vi "pulse_distribute_tester.vi"() -> ()   [LabVIEW 2021]
uses:
  <instrlib>/_niInstr/Basic Elements/v1/FPGA/niInstr Basic Elements v1 FPGA.lvlib
  <instrlib>/_niInstr/Basic Elements/v1/FPGA/Private/Count Up U64.vi
  CTL/mode_type.ctl
  pdw.ctl
  <instrlib>/_niInstr/DSP/v1/Shared/Public/IQ Data.ctl
  <instrlib>/_niInstr/DSP/v1/Shared/niInstr DSP v1 Shared.lvlib
panel:
  in  "bigger then":i32
  in  "num of loops":i32
  out "Waveform Graph":i16[][](graph)
  out "pulses read":u64=36
  in  "stop":bool
  out "output cluster":T1 {"I" format="%#_6f"}
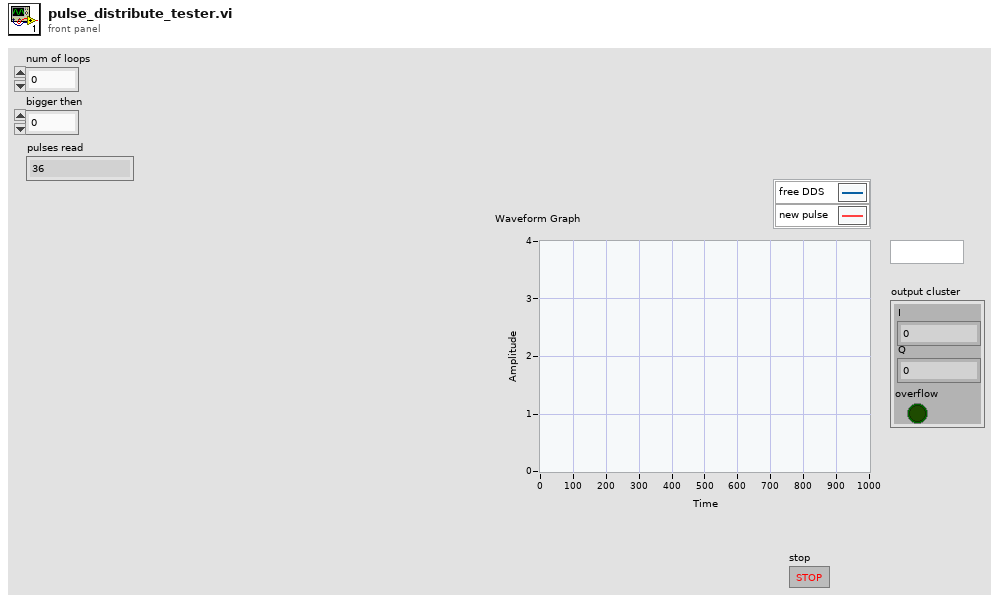
[diagram p1: front panel]
types:
  T1 = typedef "niInstr DSP v1 Shared.lvlib/IQ Data.ctl" = cluster{"I":fxp<+/-,18,1>, "Q":fxp<+/-,18,1>, "overflow":bool}
  T2 = typedef "pdw.ctl" = cluster{"PW":u32, "frequency shift":fxp<+/-,48,0>, "amp":fxp<+/-,18,1>, "mode type":T3, "mode depth":u32, "mode filter":u8, "phase shift":fxp<+/-,16,1>, "pulse shape filter":u8}
  T3 = typedef "mode_type.ctl" = enum8{"CW", "NC - CW", "NC - cw", "LFM", "BPSK", "QPSK"}
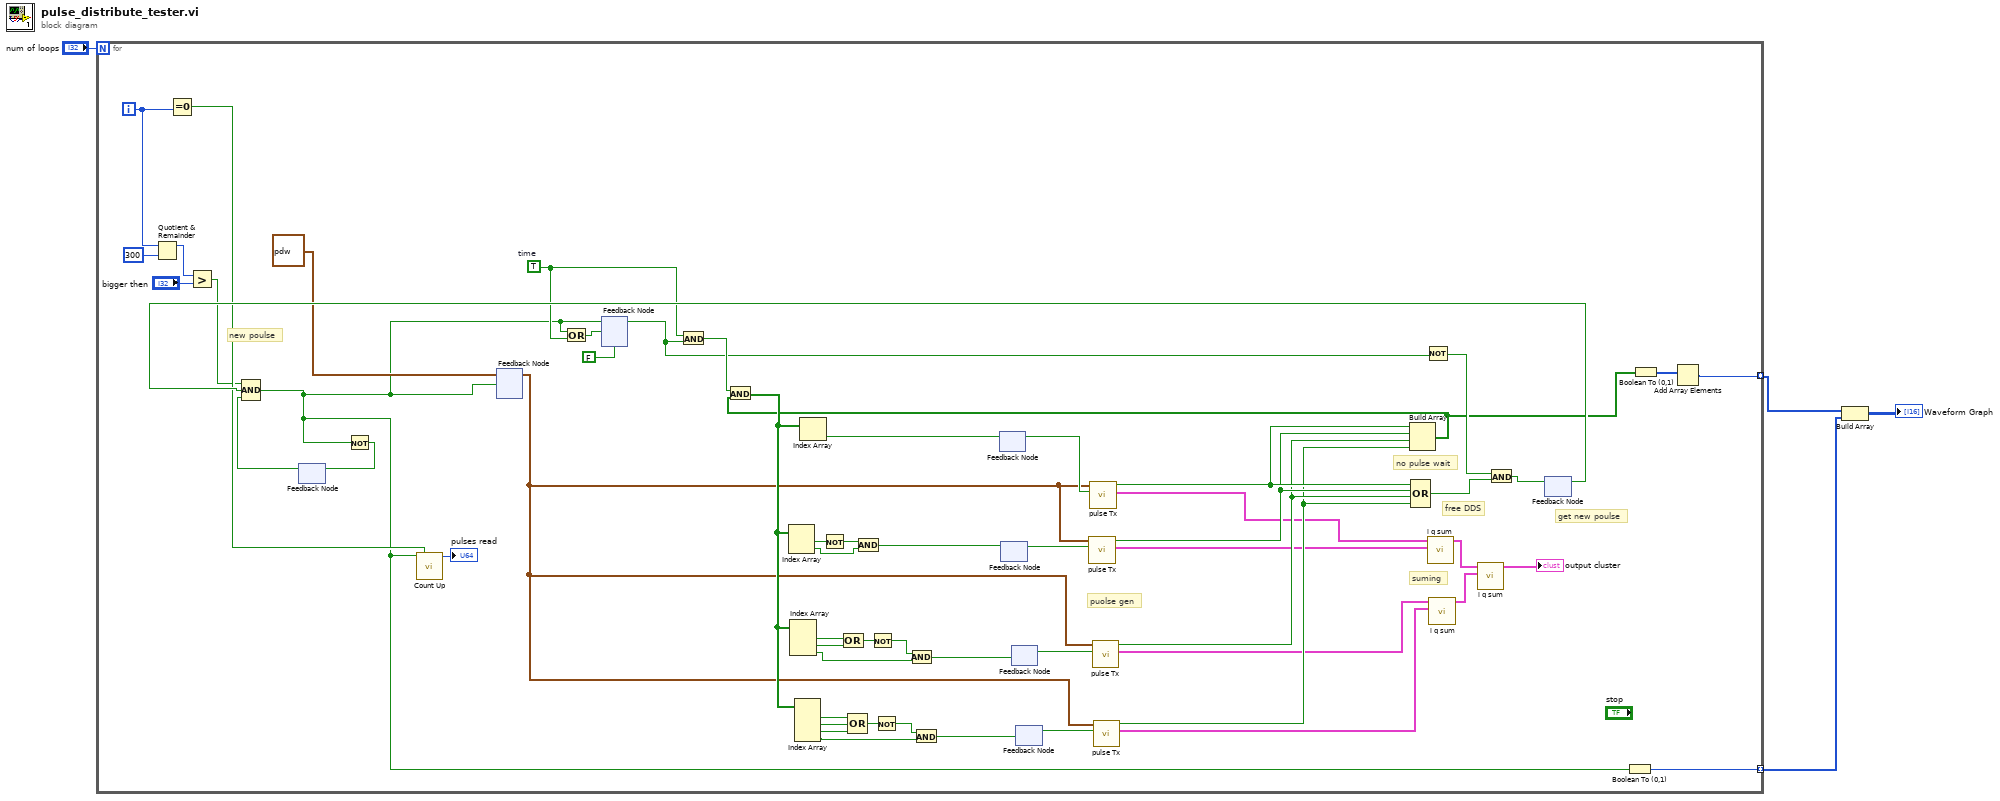
[diagram p0: block diagram]
diagram:
  n1 = for {
    N: "num of loops" -> [_]
    tunnel: [w13] -> w3 mode=indexing
    tunnel: [w10] -> w4 mode=indexing
    i -> [w9]
    w18 = TRUE  # time
    # "new poulse"
    # "suming"
    # "puolse gen"
    # "get new poulse"
    # "no pulse wait"
    # "free DDS"
    n2 = Quotient & Remainder(x=w9, y=300) -> (x-y*floor(x/y)=w7:i32)  [unwired: 1 out]
    n3 = Equal To 0?(x=w9) -> (x = 0?=w21:bool)
    n4 = Greater?(x=w7, y="bigger then") -> (0:w5:bool)
    n5 = feedback #1() -> (w23:bool)  [unwired: 1 in]
    n6 = feedback #2() -> (w15:T2)  [unwired: 1 in]
    n7 = feedback #3(FALSE ("Output Valid")) -> (w17:bool)
    n8 = And(x=w18, y=w17) -> (x .and. y?=w42:bool)
    n9 = feedback #4() -> (w31:bool)  [unwired: 1 in]
    n10 = feedback #5() -> (w53:bool)  [unwired: 1 in]
    n11 = feedback #6() -> (w52:bool)  [unwired: 1 in]
    n12 = feedback #7() -> (w50:bool)  [unwired: 1 in]
    n13 = call "pulse Tx.vi"("take it!"=w53, "Cluster"=w15) -> ("data out"=w37:T1, "free dds"=w62:bool)  [unwired: 5 in, 3 out]
    n14 = call "pulse Tx.vi"("take it!"=w31, "Cluster"=w15) -> ("data out"=w38:T1, "free dds"=w63:bool)  [unwired: 5 in, 3 out]
    n15 = call "pulse Tx.vi"("take it!"=w52, "Cluster"=w15) -> ("data out"=w36:T1, "free dds"=w51:bool)  [unwired: 5 in, 3 out]
    n16 = call "pulse Tx.vi"("take it!"=w50, "Cluster"=w15) -> ("data out"=w35:T1, "free dds"=w43:bool)  [unwired: 5 in, 3 out]
    n17 = Build Array(w63, w62, w51, w43) -> (w12:bool[])
    n18 = And(x=w42, y=w12) -> (x .and. y?=w41:bool[])
    n19 = Index Array(array=w41) -> (element #1=w61:bool, element #2=w59:bool)  [unwired: 2 in]
    n20 = Index Array(array=w41) -> (element #1=w55:bool, element #2=w56:bool, element #3=w57:bool)  [unwired: 3 in]
    n21 = Index Array(array=w41) -> (element #1=w48:bool, element #2=w47:bool, element #3=w44:bool, element #4=w45:bool)  [unwired: 4 in]
    n22 = Index Array(array=w41) -> (element=w29:bool)  [unwired: 1 in]
    n23 = Not(x=w61) -> (.not. x?=w60:bool)
    n24 = Compound Arithmetic op=OR(w55, w56) -> (w54:bool)
    n25 = Compound Arithmetic op=OR(w48, w47, w44) -> (w49:bool)
    n26 = And(x=w60, y=w59) -> (x .and. y?=w28:bool)
    n27 = Not(x=w54) -> (.not. x?=w58:bool)
    n28 = Not(x=w49) -> (.not. x?=w46:bool)
    n29 = And(x=w58, y=w57) -> (x .and. y?=w27:bool)
    n30 = And(x=w46, y=w45) -> (x .and. y?=w26:bool)
    n31 = feedback-in #4(w29) -> ()
    n32 = feedback-in #5(w28) -> ()
    n33 = feedback-in #6(w27) -> ()
    n34 = feedback-in #7(w26) -> ()
    n35 = Compound Arithmetic op=OR(w63, w62, w51, w43) -> (w39:bool)
    n36 = Not(x=w17) -> (.not. x?=w40:bool)
    n37 = call "i q sum.vi"(10:"data in"=w37, 11:"data in"=w38) -> ("output cluster"=w34:T1)  [unwired: 8 in, 1 out]
    n38 = call "i q sum.vi"(10:"data in"=w35, 11:"data in"=w36) -> ("output cluster"=w33:T1)  [unwired: 8 in, 1 out]
    n39 = call "i q sum.vi"(10:"data in"=w33, 11:"data in"=w34) -> ("output cluster"=→"output cluster":T1)  [unwired: 8 in, 1 out]
    n40 = And(x=w40, y=w39) -> (x .and. y?=w30:bool)
    n41 = feedback-in #8(w30) -> ()
    n42 = feedback #8() -> (w24:bool)  [unwired: 1 in]
    n43 = Compound Arithmetic op=AND(w5, w24, w23) -> (w14:bool)
    n44 = Not(x=w14) -> (.not. x?=w25:bool)
    n45 = feedback-in #1(w25) -> ()
    n46 = call-poly <instrlib>:"Count Up.vi"("increment"=w14, "reset"=w21) -> ("count out"=→"pulses read":u64)  [unwired: 13 in]
    n47 = feedback-in #2(T2 {"PW"=100, "frequency shift"=0.10000000000000142, "amp"=0.29998779296875, "mode type"=enum."CW", "mode depth"=0, "mode filter"=0, "phase shift"=0.0, "pulse shape filter"=6} ("Cluster"), w14) -> ()
    n48 = Or(x=w14, y=w18) -> (x .or. y?=w19:bool)
    n49 = feedback-in #3(w14, w19) -> ()
    n50 = Boolean To (0,1)(Boolean=w14) -> (0, 1=w13:i16)
    n51 = Boolean To (0,1)(Boolean=w12) -> (0, 1=w11:i16[])
    n52 = Add Array Elements(numeric array=w11) -> (sum=w10:i16)
  }
  n53 = Build Array(w4, w3) -> (→"Waveform Graph":i16[][])
